vi "PloymorphicTest.vi"(10 "B":sgl, 11 "A":sgl) -> (2 "beta":sgl, 3 "alpha":sgl)   [LabVIEW 2015]
uses:
  ABCtoAlphaBeta_2PhasePowerInvariant_src.vi
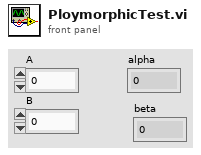
[diagram p1: front panel]
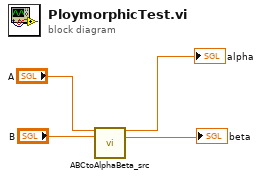
[diagram p0: block diagram]
diagram:
  n1 = call-poly "ABCtoAlphaBeta_src.vi"("A"="A", "B"="B") -> ("alpha"=→"alpha":sgl, "beta"=→"beta":sgl)  [unwired: 12 in]
